vi "test Fails If Not Equal And Provides The Context In The String.vi"(8 "error in (no error)":errorcluster, 11 "TestCase in":refnum<class "String Equality Test Case.lvclass">) -> (0 "error out":errorcluster, 3 "TestCase out":refnum<class "String Equality Test Case.lvclass">)   [LabVIEW 2015, in "String Equality Test Case.lvclass"]
uses:
  String Equality Test Case.lvclass
  <vilib>/addons/_JKI Toolkits/VI Tester/TestCase.llb/TestCase.lvclass
  VITAC.lvlib
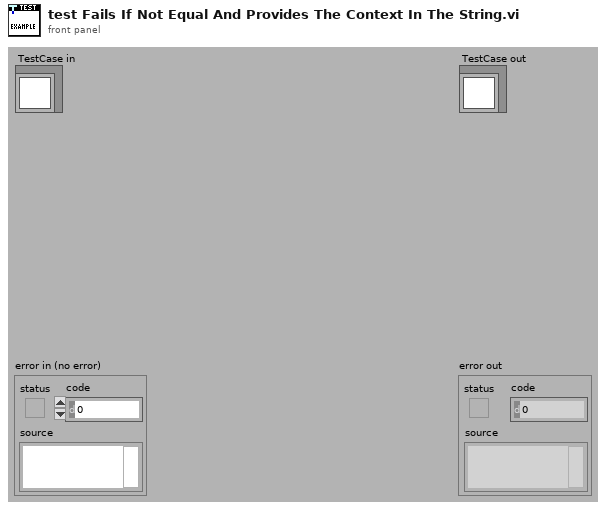
[diagram p1: front panel]
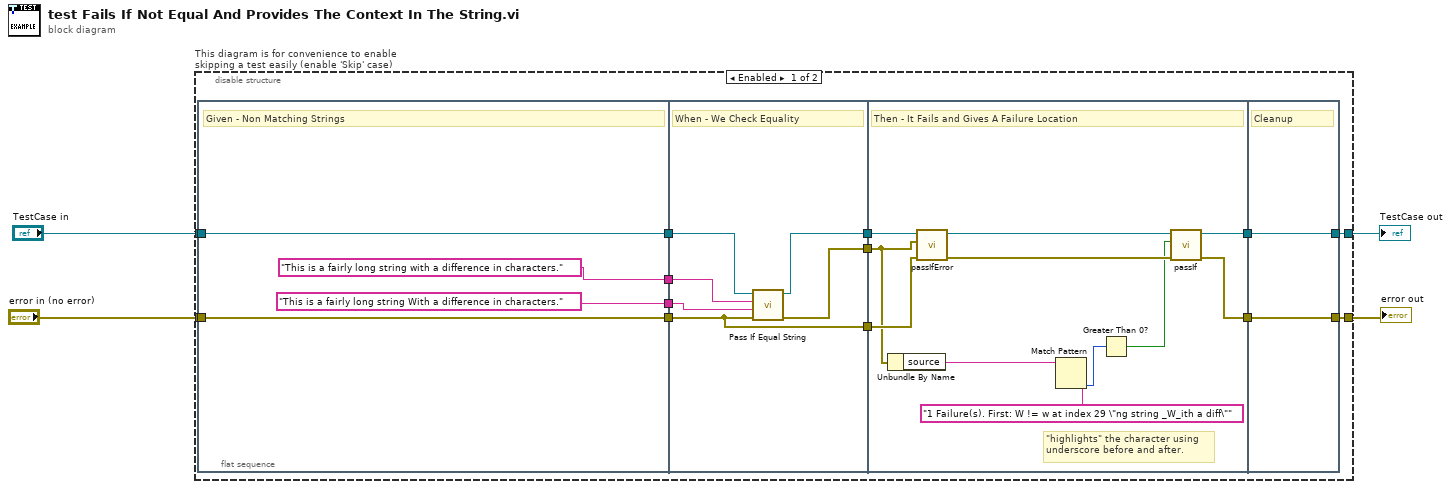
[diagram p0: block diagram]
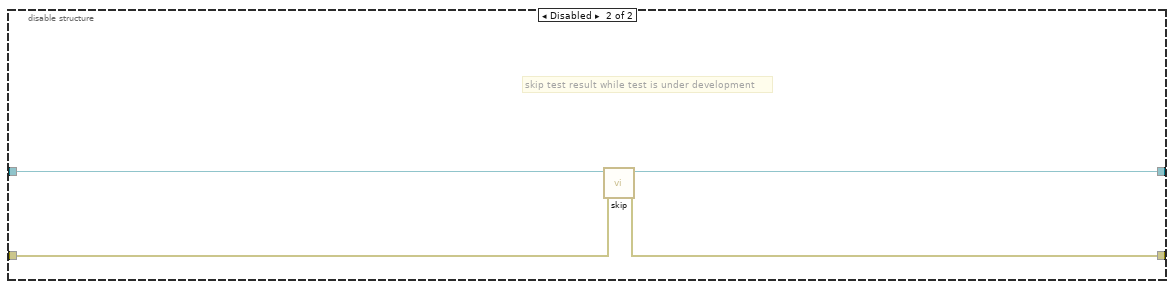
[diagram p2: hidden frame]
diagram:
  n1 = disable-structure "This diagram is for convenience to enable skipping a test easily (enable 'Skip' case)" shown="Enabled" {
    disable-tunnel: "TestCase in" -> [w17 w44]
    disable-tunnel: [w16 w42] -> w1
    disable-tunnel: [w15 w43] -> w3
    disable-tunnel: "error in (no error)" -> [w14 w41]
    frame Enabled {
      n2 = flat-sequence {
        tunnel: w14 -> [w20]
        tunnel: w17 -> [w21]
        tunnel: [w21] -> w10
        tunnel: [w20] -> w9
        tunnel: ["This is a fairly long string with a difference in characters." ("expected")] -> w8
        tunnel: ["This is a fairly long string With a difference in characters." ("expected")] -> w7
        tunnel: [w26] -> w11
        tunnel: w10 -> [w27]
        tunnel: w9 -> [w22]
        tunnel: w8 -> [w25]
        tunnel: w7 -> [w24]
        tunnel: [w23] -> w6
        tunnel: [w22] -> w5
        tunnel: [w36] -> w13
        tunnel: [w35] -> w12
        tunnel: w11 -> [w38]
        tunnel: w6 -> [w28]
        tunnel: w5 -> [w30]
        tunnel: [w39] -> w15
        tunnel: [w40] -> w16
        tunnel: w13 -> [w40]
        tunnel: w12 -> [w39]
        frame #0 {
          # "Given - Non Matching Strings"
        }
        frame #1 {
          # "When - We Check Equality"
          n3 = call "Pass If Equal String.vi"("error in (no error)"=w22, "actual"=w24, "expected"=w25, "TestCase in"=w27) -> ("error out"=w23:errorcluster, "TestCase out"=w26:refnum<class "String Equality Test Case.lvclass">)  [unwired: 6 in]
        }
        frame #2 {
          # "\"highlights\" the character using\nunderscore before and after."
          # "Then - It Fails and Gives A Failure Location"
          n4 = Unbundle By Name(w28) -> ("source"=w33:string)
          n5 = call-dynamic "passIfError.vi"("error in (no error)"=w30, "error"=w28, "TestCase in"=w38) -> ("error out"=w34:errorcluster, "TestCase out"=w37:refnum<class "String Equality Test Case.lvclass">)  [unwired: 7 in]
          n6 = Match Pattern(string=w33, regular expression="1 Failure(s). First: W != w at index 29 \"ng string _W_ith a diff\"") -> (offset past match=w31:i32)  [unwired: 1 in, 3 out]
          n7 = Greater Than 0?(x=w31) -> (x > 0?=w29:bool)
          n8 = call-dynamic "passIf.vi"("error in (no error)"=w34, "pass"=w29, "TestCase in"=w37) -> ("error out"=w35:errorcluster, "TestCase out"=w36:refnum<class "String Equality Test Case.lvclass">)  [unwired: 7 in]
        }
        frame #3 {
          # "Cleanup"
        }
      }
    }
    frame Disabled {
      # "skip test result while test is under development"
      n9 = call <vilib>:"skip.vi"("error in (no error)"=w41, "TestCase in"=w44) -> ("error out"=w43:errorcluster, "TestCase out"=w42:refnum<class "String Equality Test Case.lvclass">)  [unwired: 8 in]
    }
  }
  "error out" <- w3
  "TestCase out" <- w1
